vi "XML Script - SubVI (Refnum).vi"(0 "x":i32=-1, 1 "y":i32=-1, 2 "out":i32=-1, 4 "path (VI Refnum)":refnum<vi>, 6 "name":string, 9 "prefix (name)":string, 10 "in":i32=-1) -> (5 "name (wire source)":string, 7 "XML Script Command - SubVI":string)   [LabVIEW 2020]
panel:
  # "position"
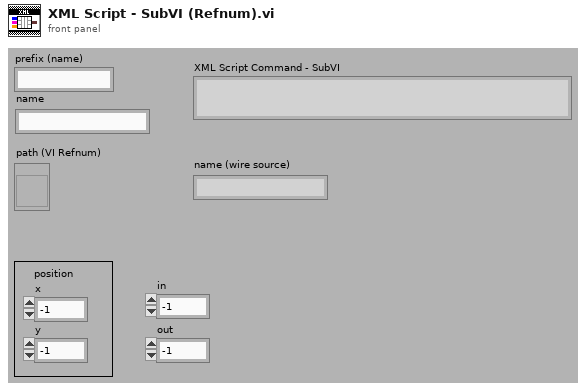
[diagram p1: front panel]
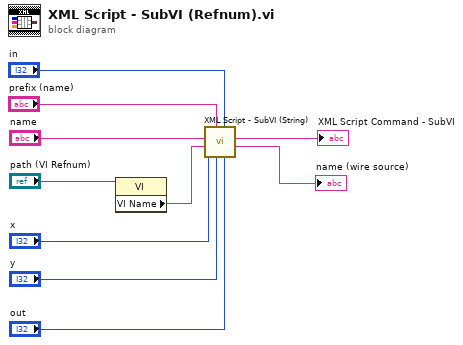
[diagram p0: block diagram]
diagram:
  n1 = property class="VI"(reference="path (VI Refnum)") -> ("VI Name"=w8:string)  [unwired: 1 in, 2 out]
  n2 = call <vilib>:"XML Script - SubVI (String).vi"("x"="x", "y"="y", "out"="out", "path"=w8, "name"="name", "prefix (name)"="prefix (name)", "in"="in") -> ("name (wire source)"=→"name (wire source)":string, "XML Script Command - SubVI"=→"XML Script Command - SubVI":string)  [unwired: 3 in]
